vi "Get IPE Diagram.vi"(11 "VI Ref":refnum<vi>) -> (3 "IPE Diagram":refnum<vi>)   [LabVIEW 2018, in "LVClassByRef.lvlib"]
uses:
  <resource>/Framework/Providers/LVClassByRef/LVClassByRef.lvlib
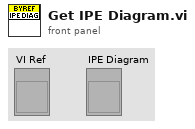
[diagram p1: front panel]
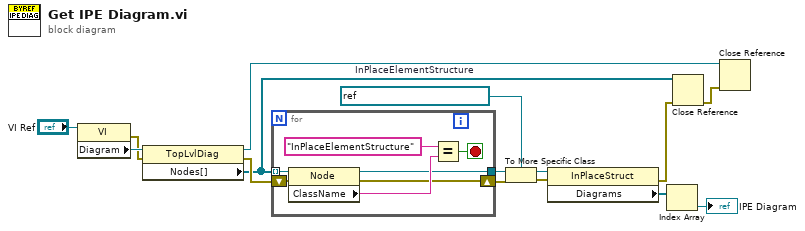
[diagram p0: block diagram]
diagram:
  w12 = refnum<vi> refnum  # InPlaceElementStructure
  n1 = property class="VI"(reference="VI Ref") -> (error out=w9:errorcluster, "Diagram"=w14:refnum<vi>)  [unwired: 1 in, 1 out]
  n2 = property class="TopLvlDiag"(reference=w14, error in=w9) -> (reference out=w1:refnum<vi>, error out=w15:errorcluster, "Nodes[]"=w6:refnum<vi>[])
  n3 = for {
    tunnel: w6 -> [w22] mode=indexing
    tunnel: [w18] -> w13
    shift-right: [w16] -> w8
    shift-left: w15 -> [w17]
    stop <- w19 stop-if-true
    n4 = property class="Node"(reference=w22, error in=w17) -> (reference out=w18:refnum<vi>, error out=w16:errorcluster, "ClassName"=w20:string)
    n5 = Equal?(x="InPlaceElementStructure", y=w20) -> (x = y?=w19:bool)
  }
  n6 = To More Specific Class(target class=w12, reference=w13, error in=w8) -> (specific class reference=w11:refnum<vi>, error out=w7:errorcluster)
  n7 = property class="InPlaceStruct"(reference=w11, error in=w7) -> (error out=w5:errorcluster, "Diagrams"=w10:refnum<vi>[])  [unwired: 1 out]
  n8 = Index Array(array=w10) -> (element=→"IPE Diagram":refnum<vi>)  [unwired: 1 in]
  n9 = Close Reference(reference=w6, error in (no error)=w5) -> (error out=w2:errorcluster)
  n10 = Close Reference(reference=w1, error in (no error)=w2) -> ()  [unwired: 1 out]
